vi "AppMenuSelection.vi"(8 "error in (no error)":errorcluster, 10 "Menu Selection in":string, 11 "FPGADMAChannelData in":refnum<class "FPGADMAChannelData.lvclass">) -> (0 "error out":errorcluster, 1 "New Message":string, 2 "Menu Selection out":string, 3 "FPGADMAChannelData out":refnum<class "FPGADMAChannelData.lvclass">)   [LabVIEW 2013, in "FPGADMAChannelData.lvclass"]
doc: "Processes the action related to the application level menu selection. For instance used when the user chooses \"File->Save\""
uses:
  FPGADMAChannelData.lvclass
  FPGADMAChannelData.lvclass/FPGADMAChannelData.ctl
  xCE/xceRootNode/xceRootNode.lvclass
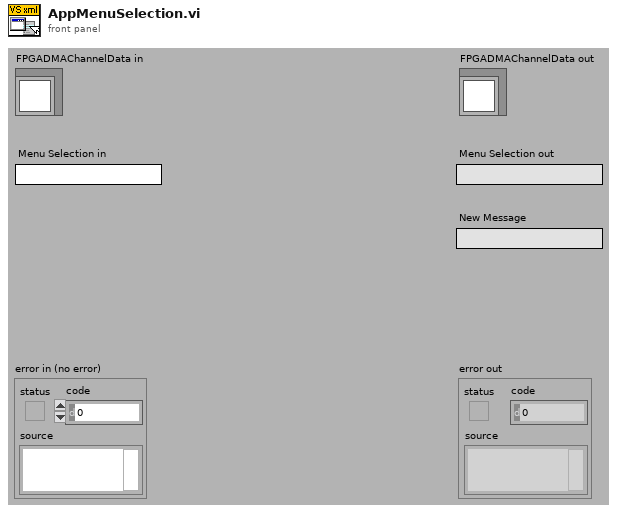
[diagram p1: front panel]
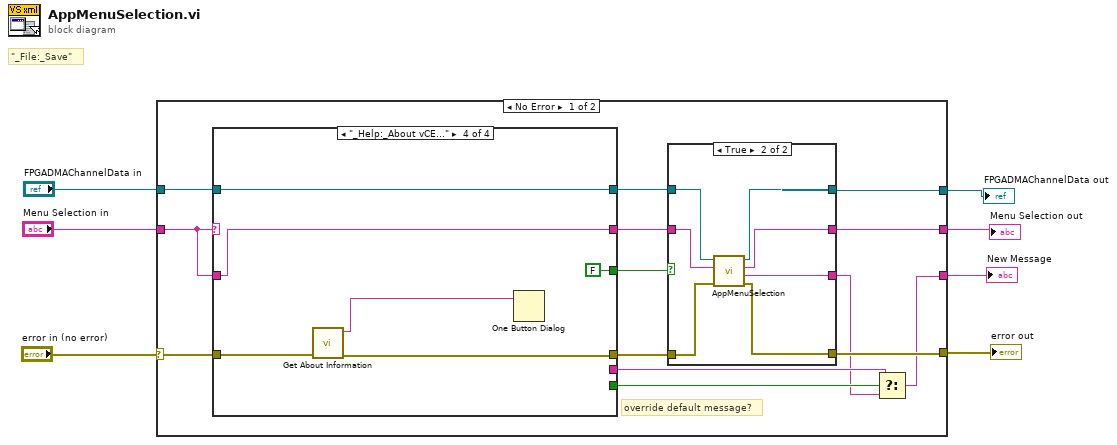
[diagram p0: block diagram]
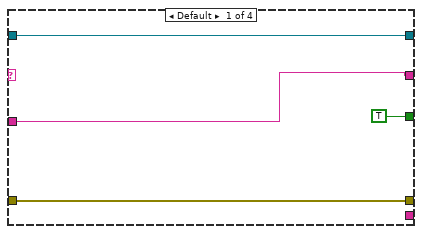
[diagram p3: hidden frame]
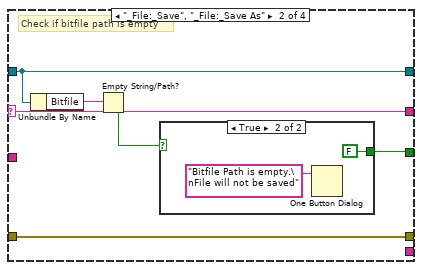
[diagram p4: hidden frame]
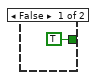
[diagram p5: hidden frame]
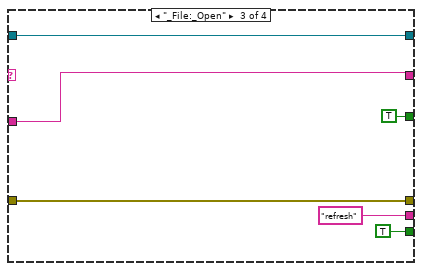
[diagram p6: hidden frame]
diagram:
  # "\"_File:_Save\""
  n1 = case shown="No Error" "error in (no error)" {
    selector: "error in (no error)" -> [w21 w57]
    tunnel: "Menu Selection in" -> [w12 w58]
    tunnel: "FPGADMAChannelData in" -> [w20 w59]
    tunnel: [w18 w59] -> w4
    tunnel: [w14 w58] -> w3
    tunnel: [w8 _] -> w2
    tunnel: [w13 w57] -> w1
    frame No Error {
      # "override default message?"
      n2 = case shown="\"_Help:_About vCE...\"" w12 {
        selector: w12 -> [_ w39 _ _]
        tunnel: w21 -> [w34 w36 w47 w53]
        tunnel: w20 -> [w35 w40 w50 w54]
        tunnel: [w35 w40 w50 w54] -> w19
        tunnel: [w34 w36 w47 w51] -> w17
        tunnel: [TRUE w37 TRUE FALSE] -> w16
        tunnel: [w32 w39 w48 w55] -> w15
        tunnel: w12 -> [w32 _ w48 w55]
        tunnel: [_ _ TRUE _] -> w11
        tunnel: [_ _ "refresh" _] -> w10
        frame Default {
        }
        frame "_File:_Save", "_File:_Save As" {
          # "Check if bitfile path is empty"
          n3 = Unbundle By Name(w40) -> ("Bitfile"=w41:string)
          n4 = Empty String/Path?(string/path=w41) -> (empty?=w38:bool)
          n5 = case shown="True" w38 {
            tunnel: [TRUE FALSE] -> w37
            frame False {
            }
            frame True {
              n6 = One Button Dialog(message="Bitfile Path is empty.\nFile will not be saved") -> ()  [unwired: 1 in, 1 out]
            }
          }
        }
        frame "_File:_Open" {
        }
        frame "_Help:_About vCE..." {
          n7 = call "Get About Information.vi"("error in (no error)"=w53) -> ("error out"=w51:errorcluster, "About vCE text Out"=w52:string)  [unwired: 9 in]
          n8 = One Button Dialog(message=w52) -> ()  [unwired: 1 in, 1 out]
        }
      }
      n9 = case shown="True" w16 {
        tunnel: w19 -> [w24 w31]
        tunnel: [w24 w30] -> w18
        tunnel: w17 -> [w22 w29]
        tunnel: w15 -> [w23 w28]
        tunnel: [w23 w27] -> w14
        tunnel: [_ w26] -> w9
        tunnel: [w22 w25] -> w13
        frame False {
        }
        frame True {
          n10 = call-parent "AppMenuSelection.vi"("error in (no error)"=w29, "Menu Selection in"=w28, "xceRootNode in"=w31) -> ("error out"=w25:errorcluster, "New Message"=w26:string, "Menu Selection out"=w27:string, "xceRootNode out"=w30:refnum<class "FPGADMAChannelData.lvclass">)  [unwired: 5 in]
        }
      }
      n11 = Select(t=w10, s=w11, f=w9) -> (s? t:f=w8:string)
    }
    frame Error {
    }
  }
  "error out" <- w1
  "FPGADMAChannelData out" <- w4
  "Menu Selection out" <- w3
  "New Message" <- w2
